vi "Create ERROR msg.vi"(8 "error in":errorcluster, 11 "Error Request":T1 {"Message Type" items=["HELLO"=1, "WELCOME"=2, "ABORT"=3, "GOODBYE"=6, "ERROR"=8, "PUBLISH"=16, "PUBLISHED"=17, "SUBSCRIBE"=32, "SUBSCRIBED"=33, "UNSUBSCRIBE"=34, "UNSUBSCRIBED"=35, "EVENT"=36, "CALL"=48, "RESULT"=59, "REGISTER"=64, "REGISTERED"=65, "UNREGISTER"=66, "UNREGISTERED"=67, "INVOCATION"=68, "YIELD"=70]}) -> (0 "error out":errorcluster, 3 "String":string)   [LabVIEW 2020, in "wamplv.lvlib" / "WAMP Client.lvclass"]
uses:
  WAMP Client.lvclass
  TypeDef/Error Request.ctl
  API/TypeDefs/WAMP error.ctl
  Private/TypeDefs/WAMP Message Codes.ctl
  WAMP Client.lvclass/WAMP Client.ctl
  Private/Utils/Utils.lvclass
  wamplv.lvlib
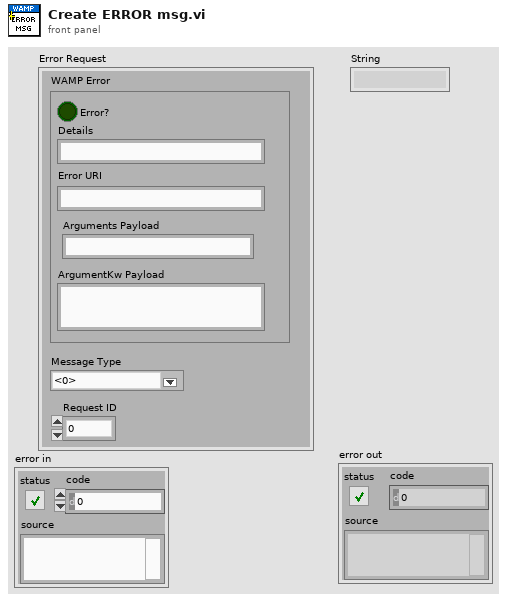
[diagram p1: front panel]
types:
  T1 = typedef "wamplv.lvlib/WAMP Client.lvclass/Error Request.ctl" = cluster{"WAMP Error":T2, "Message Type":T3, "Request ID":u64}
  T2 = typedef "wamplv.lvlib/WAMP Client.lvclass/WAMP error.ctl" = cluster{"Details":string, "ArgumentKw Payload":string, "Error?":bool, "Error URI":string, "Arguments Payload":string}
  T3 = typedef "wamplv.lvlib/WAMP Message Codes.ctl" = u16
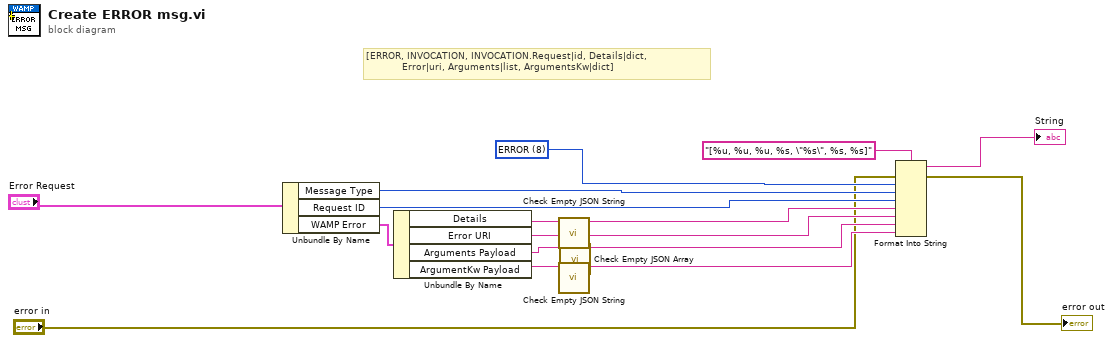
[diagram p0: block diagram]
diagram:
  w5 = T3 8 items=["HELLO"=1, "WELCOME"=2, "ABORT"=3, "GOODBYE"=6, "ERROR"=8, "PUBLISH"=16, "PUBLISHED"=17, "SUBSCRIBE"=32, "SUBSCRIBED"=33, "UNSUBSCRIBE"=34, "UNSUBSCRIBED"=35, "EVENT"=36, "CALL"=48, "RESULT"=59, "REGISTER"=64, "REGISTERED"=65, "UNREGISTER"=66, "UNREGISTERED"=67, "INVOCATION"=68, "YIELD"=70] ("Message Codes")
  # "[ERROR, INVOCATION, INVOCATION.Request|id, Details|dict,\n            Error|uri, Arguments|list, ArgumentsKw|dict]"
  n1 = Unbundle By Name("Error Request") -> ("Message Type"=w6:T3, "Request ID"=w7:u64, "WAMP Error"=w8:T2)
  n2 = Unbundle By Name(w8) -> ("Details"=w10:string, "Error URI"=w9:string, "Arguments Payload"=w15:string, "ArgumentKw Payload"=w12:string)
  n3 = call "Check Empty JSON String.vi"("JSON in"=w10) -> ("JSON out"=w11:string)  [unwired: 10 in]
  n4 = call "Check Empty JSON String.vi"("JSON in"=w12) -> ("JSON out"=w13:string)  [unwired: 10 in]
  n5 = call "Check Empty JSON Array.vi"("JSON in"=w15) -> ("JSON out"=w16:string)  [unwired: 10 in]
  n6 = Format Into String(format string="[%u, %u, %u, %s, \"%s\", %s, %s]" ("element"), error in="error in", w5, w6, w7, w11, w9, w16, w13) -> (resulting string=→"String":string, error out=→"error out":errorcluster)  [unwired: 1 in]
